vi "Get New Level.vi"(8 "error in (no error)":errorcluster, 11 "Cooler in":refnum<class "Cooler.lvclass">) -> (0 "error out":errorcluster, 2 "Level":dbl, 3 "Cooler out":refnum<class "Cooler.lvclass">)   [LabVIEW 2025, in "Cooler.lvlib" / "Cooler.lvclass"]
doc: "Child classes should not need to override this VI. If they do, they must invoke the Call Parent node."
uses:
  Cooler.lvclass
  Cooler.lvclass/Cooler.ctl
  Cooler Controller/Update Current Temperature Msg/Update Current Temperature Msg.lvclass/Update Current Temperature Msg.ctl
  <vilib>/ActorFramework/Message Enqueuer/Message Enqueuer.lvclass/Message Enqueuer.ctl
  <vilib>/ActorFramework/Message Enqueuer/Enqueue.vi
  Cooler Controller/Update Current Temperature Msg/Update Current Temperature Msg.lvclass
  C:/Program Files/National Instruments/LabVIEW 2025/vi.lib/ActorFramework/Message/Message.lvclass
  <vilib>/ActorFramework/Message Priority Queue/Priority Enqueue.vi
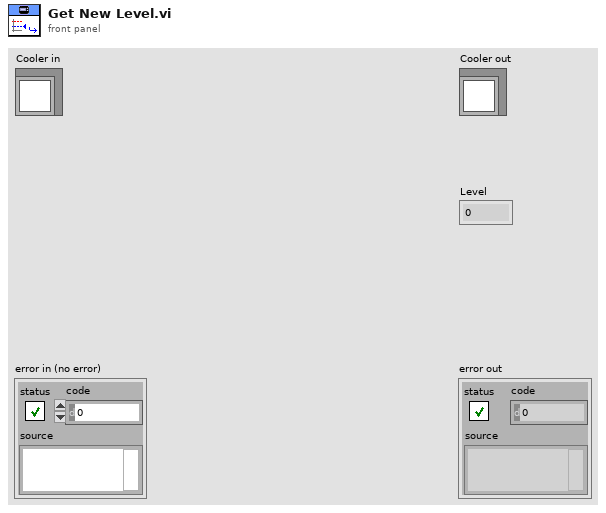
[diagram p1: front panel]
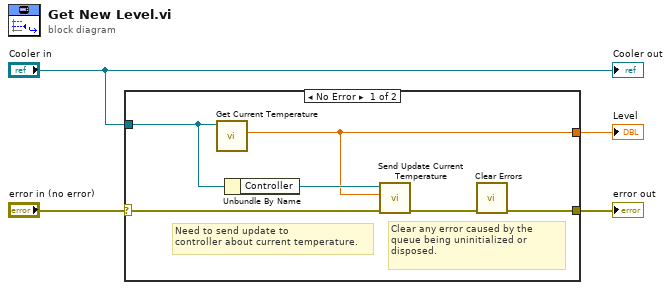
[diagram p0: block diagram]
diagram:
  n1 = case shown="No Error" "error in (no error)" {
    selector: "error in (no error)" -> [w7 w11]
    tunnel: "Cooler in" -> [w10 _]
    tunnel: [w8 _] -> w3
    tunnel: [w5 w11] -> w2
    frame No Error {
      # "Clear any error caused by the queue being uninitialized or disposed."
      # "Need to send update to \ncontroller about current temperature."
      n2 = call-dynamic "Get Current Temperature.vi"("Cooler in"=w10) -> ("Level"=w8:dbl)  [unwired: 9 in, 1 out]
      n3 = Unbundle By Name(w10) -> ("Controller"=w9:refnum<class "Message Enqueuer.lvclass">)
      n4 = call "Send Update Current Temperature.vi"("error in (no error)"=w7, "Current Temperature"=w8, "Message Enqueuer"=w9) -> ("error out"=w6:errorcluster)  [unwired: 8 in]
      n5 = call <vilib>:"Clear Errors.vi"("error in (no error)"=w6) -> ("error out"=w5:errorcluster)  [unwired: 5 in, 1 out]
    }
    frame Error {
    }
  }
  "error out" <- w2
  "Level" <- w3
  "Cooler out" <- "Cooler in"
